vi "SphereStripRim.vi"(6 "number of points":i32=200, 10 "Ducer":cluster{"radius":dbl, "h":dbl, "w":dbl} {"radius" format="%.2f"; "w" format="%.2f"; "h" format="%.2f"}) -> (0 "rim points":dbl[][](array[numeric]) format="%.2f")   [LabVIEW 2022 SP3]
panel:
  # "Find co-ordinates of strip rim. Use normal XYZ with strip center on -Y axis and look in -Y direction. Start strip at +X,+Z, go down, right, up, left and back to start position."
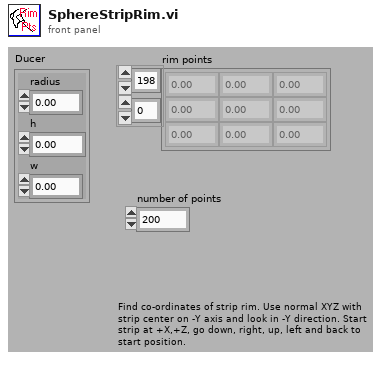
[diagram p1: front panel]
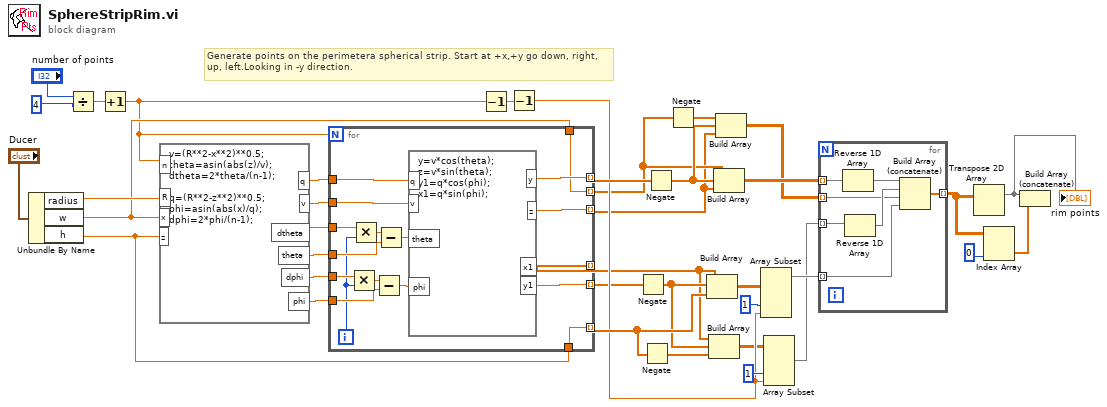
[diagram p0: block diagram]
diagram:
  # "Generate points on the perimetera spherical strip. Start at +x,+y go down, right, up, left.Looking in -y direction."
  n1 = Unbundle By Name("Ducer") -> ("radius"=w38:dbl, "w"=w36:dbl, "h"=w35:dbl)
  n2 = Divide(x="number of points", y=4) -> (x/y=w5:dbl)
  n3 = Increment(x=w5) -> (x+1=w3:dbl)
  n4 = formula code="v=(R**2-x**2)**0.5;\ntheta=asin(abs(z)/v);\ndtheta=2*theta/(n-1);\n\nq=(R**2-z**2)**0.5;\nphi=asin(abs(x)/q);\ndphi=2*phi/(n-1);"("R"=w38, "x"=w36, "n"=w3, "z"=w35) -> ("v"=w32:dbl, "dtheta"=w34:dbl, "theta"=w33:dbl, "q"=w29:dbl, "dphi"=w31:dbl, "phi"=w30:dbl)
  n5 = for {
    N: w3 -> [_]
    tunnel: [w49] -> w15 mode=indexing
    tunnel: [w55] -> w37 mode=indexing
    tunnel: [w54] -> w14 mode=indexing
    tunnel: w34 -> [w53]
    tunnel: w33 -> [w51]
    tunnel: w36 -> [w49]
    tunnel: w32 -> [w48]
    tunnel: w31 -> [w40]
    tunnel: w30 -> [w46]
    tunnel: [w44] -> w13 mode=indexing
    tunnel: [w43] -> w12 mode=indexing
    tunnel: w35 -> [w42]
    tunnel: [w42] -> w26 mode=indexing
    tunnel: w29 -> [w41]
    i -> [w39]
    n6 = Multiply(x=w40, y=w39) -> (x*y=w47:dbl)
    n7 = Multiply(x=w53, y=w39) -> (x*y=w52:dbl)
    n8 = Subtract(x=w47, y=w46) -> (x-y=w45:dbl)
    n9 = Subtract(x=w52, y=w51) -> (x-y=w50:dbl)
    n10 = formula code="y=v*cos(theta);\nz=v*sin(theta);\ny1=q*cos(phi);\nx1=q*sin(phi);"("v"=w48, "theta"=w50, "q"=w41, "phi"=w45) -> ("y"=w55:dbl, "z"=w54:dbl, "x1"=w44:dbl, "y1"=w43:dbl)
  }
  n11 = Decrement(x=w3) -> (x-1=w28:dbl)
  n12 = Decrement(x=w28) -> (x-1=w17:dbl)
  n13 = Negate(x=w12) -> (-x=w19:dbl[])
  n14 = Negate(x=w26) -> (-x=w20:dbl[])
  n15 = Negate(x=w37) -> (-x=w22:dbl[])
  n16 = Negate(x=w15) -> (-x=w23:dbl[])
  n17 = Build Array(w13, w19, w26) -> (w11:dbl[][])
  n18 = Build Array(w13, w19, w20) -> (w10:dbl[][])
  n19 = Build Array(w15, w22, w14) -> (w27:dbl[][])
  n20 = Build Array(w23, w22, w14) -> (w21:dbl[][])
  n21 = Array Subset(array=w11, index (col)=1, length (col)=w17) -> (w24:dbl[][])  [unwired: 2 in]
  n22 = Array Subset(array=w10, index (col)=1, length (col)=w17) -> (w16:dbl[][])  [unwired: 2 in]
  n23 = for {
    tunnel: w27 -> [w61] mode=indexing
    tunnel: w24 -> [w56] mode=indexing
    tunnel: w21 -> [w57] mode=indexing
    tunnel: w16 -> [w59] mode=indexing
    tunnel: [w62] -> w7 mode=indexing
    n24 = Reverse 1D Array(array=w61) -> (reversed array=w60:dbl[])
    n25 = Reverse 1D Array(array=w59) -> (reversed array=w58:dbl[])
    n26 = Build Array (concatenate)(w60, w58, w57, w56) -> (w62:dbl[])
  }
  n27 = Transpose 2D Array(2D array=w7) -> (transposed array=w2:dbl[][])
  "rim points" <- w2
  n28 = Index Array(array=w7, index (col)=0) -> (element=w9:dbl[])  [unwired: 1 in]
  n29 = Build Array (concatenate)(w2, w9) -> ()  [unwired: 1 out]
